vi "GEN_Set Bool Color.vi"(9 "alarm":bool, 10 "stop":bool, 11 "ref":refnum<vi>) -> ()   [LabVIEW 2016]
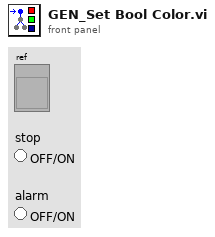
[diagram p1: front panel]
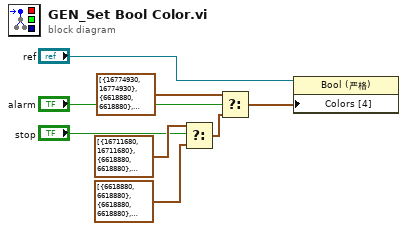
[diagram p0: block diagram]
diagram:
  n1 = Select(t=cluster{u32, u32}[] [{16711680, 16711680}, {6618880, 6618880}, {8354569, 8354569}, {6618880, 6618880}] ("颜色[4] 2"), s="stop", f=cluster{u32, u32}[] [{6618880, 6618880}, {6618880, 6618880}, {8354569, 8354569}, {6618880, 6618880}] ("颜色[4] 2")) -> (s? t:f=w7:cluster{u32, u32}[])
  n2 = Select(t=cluster{u32, u32}[] [{16774930, 16774930}, {6618880, 6618880}, {8354569, 8354569}, {6618880, 6618880}] ("颜色[4] 2"), s="alarm", f=w7) -> (s? t:f=w8:cluster{u32, u32}[])
  n3 = property on="属性节点" class="Bool (严格)"(reference="ref", "Colors [4]"=w8) -> ()  [unwired: 1 in, 2 out]
